vi "GetDH.vi"(8 "error in (no error)":errorcluster, 10 "BodyID":i32, 11 "Bodies.lvclass In":refnum<class "Bodies.lvclass">) -> (0 "error out":errorcluster, 2 "Transfer Matrix":T1, 3 "Bodies.lvclass Out":refnum<class "Bodies.lvclass">)   [LabVIEW 2012, in "Bodies.lvclass"]
uses:
  Bodies.lvclass
  <vilib>/Analysis/Matrix/Datatypes/RealMatrix.ctl
  Bodies.lvclass/Bodies.ctl
  <vilib>/Analysis/Matrix/Numeric/Conversions/Array To Matrix - RA2.vi
  <vilib>/Analysis/Matrix/NI_Matrix.lvlib
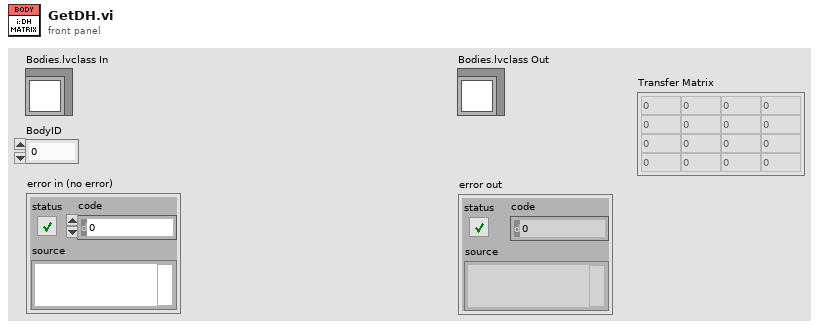
[diagram p1: front panel]
types:
  T1 = typedef "NI_Matrix.lvlib/RealMatrix.ctl" = dbl[][]
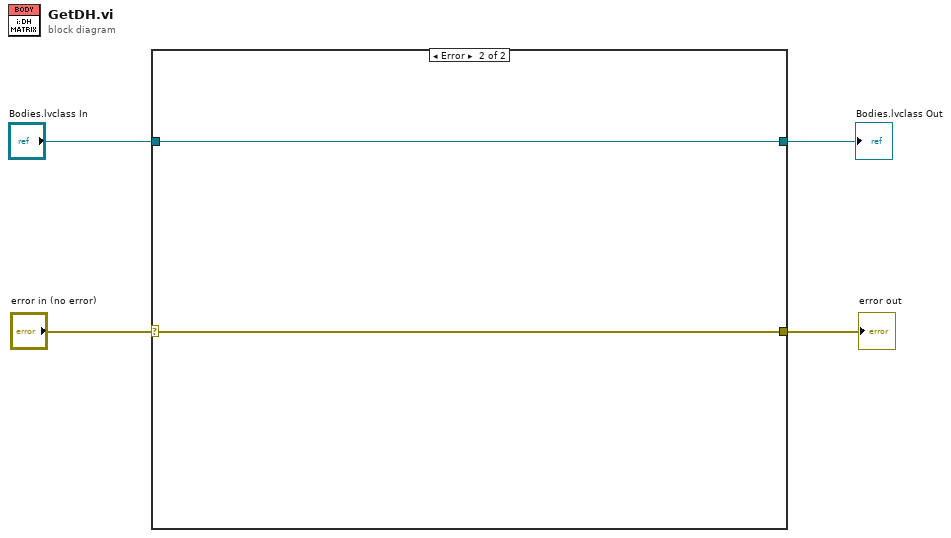
[diagram p0: block diagram]
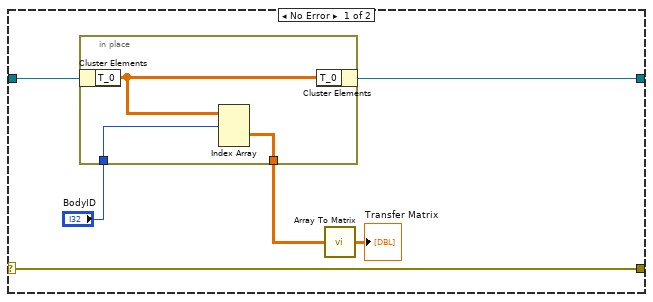
[diagram p2: hidden frame]
diagram:
  n1 = case shown="Error" "error in (no error)" {
    selector: "error in (no error)" -> [w5 w14]
    tunnel: "Bodies.lvclass In" -> [w10 w15]
    tunnel: [w6 w15] -> w2
    tunnel: [w5 w14] -> w1
    frame No Error {
      n2 = in-place {
        in-place-border: "BodyID" -> [w13]
        in-place-border: [w12] -> w8
        n3 = in-place-cluster #1(w10) -> ("T_0"=w11:dbl[][][])
        n4 = Index Array(array=w11, index (dim 0)=w13) -> (element=w12:dbl[][])  [unwired: 2 in]
        n5 = in-place-cluster #1("T_0"=w11) -> (w6:refnum<class "Bodies.lvclass">)
      }
      n6 = call-poly <vilib>:"Array To Matrix.vi"("Real 2D Array"=w8) -> ("Real Matrix"=→"Transfer Matrix":T1)
    }
    frame Error {
    }
  }
  "error out" <- w1
  "Bodies.lvclass Out" <- w2
